vi "LUCS001RT_GPS_RS232_ReadxB5.vi"(8 "error in":errorcluster, 9 "FPGA VI Reference":refnum<k20>) -> (0 "error out":errorcluster, 1 "FPGA VI Reference Out":refnum<k20>, 3 "TimedOut?":bool, 5 "Numeric":u8 format="%01x")   [LabVIEW 2020]
uses:
  <vilib>/rvi/interface/nirviMethod/nirviMethod.xnode
  sbRIO-9612/SourceCodeFPGA/LUCS002FPGA_Main.vi
  SourceCode_Host/SourceCode_Host/FPGA Bitfiles/LUCS002h.lvproj_FPGA Target_LUCS002FPGA_Main.vi.lvbit
  <vilib>/FPGAPlugInAG/sbRIO-9612/niLvFpga_ReadFifo_sbRIO-9612.vi
  <vilib>/rvi/errors/niLvFpgaMergeErrorWithErrorCode.vi
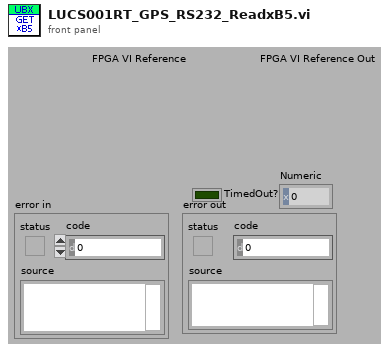
[diagram p1: front panel]
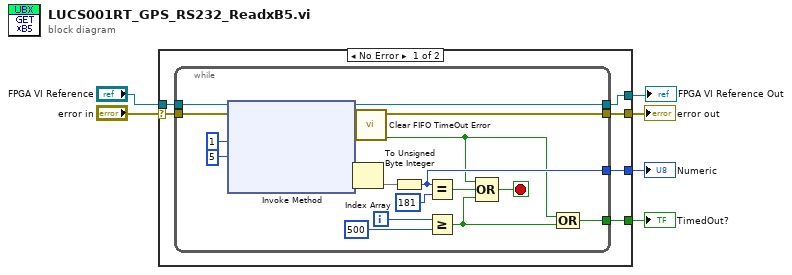
[diagram p0: block diagram]
diagram:
  n1 = case shown="No Error" "error in" {
    selector: "error in" -> [w8 w31]
    tunnel: [w12 _] -> w6
    tunnel: [w11 _] -> w1
    tunnel: [w10 w31] -> w5
    tunnel: "FPGA VI Reference" -> [w9 _]
    tunnel: [w7 _] -> w3
    frame No Error {
      n2 = while {
        tunnel: w8 -> [w30]
        tunnel: w9 -> [w29]
        tunnel: [w16] -> w10
        tunnel: [w22] -> w11
        tunnel: [w13] -> w12
        tunnel: [w18] -> w7
        i -> [w21]
        stop <- w19 stop-if-true
        n3 = xnode "Invoke Method"("FPGA VI Reference In"=w29, "error in"=w30, "Number of Elements"=u32 1, "Timeout (ms)"=5) -> ("FPGA VI Reference Out"=w22:refnum<k20>, "error out"=w17:errorcluster, "Data"=w26:void[])  [unwired: 1 out]
        n4 = Index Array(array=w26) -> (element=w25)  [unwired: 1 in]
        n5 = call "Clear FIFO TimeOut Error.vi"("error in (no error)"=w17) -> ("TimedOut"=w15:bool, "error out"=w16:errorcluster)  [unwired: 9 out]
        n6 = To Unsigned Byte Integer(number=w25) -> (unsigned 8bit integer=w18:u8)
        n7 = Equal?(x=w18, y=u8 181 ("element")) -> (x = y?=w23:bool)
        n8 = Greater Or Equal?(x=w21, y=500) -> (x >= y?=w14:bool)
        n9 = Compound Arithmetic op=OR(w15, w23, w14) -> (w19:bool)
        n10 = Compound Arithmetic op=OR(w15, w14) -> (w13:bool)
      }
    }
    frame Error {
    }
  }
  "TimedOut?" <- w6
  "error out" <- w5
  "Numeric" <- w3
  "FPGA VI Reference Out" <- w1
